vi "Rotation_GetSin.vi"(11 "in ROTATION":T1={"VALUE"=0.0, "COS"=1.0, "SIN"=0.0}) -> (3 "SINE":dbl)   [LabVIEW 2019, in "Trajectory_Library.lvlib"]
doc: "Returns the sine of the rotation.\n\nParameters:\n - in ROTATION - This ROTATION data structure\n\nReturns:\n - Sine of the ROTATAION"
uses:
  Trajectory_Library.lvlib
  ROTATION2D.ctl
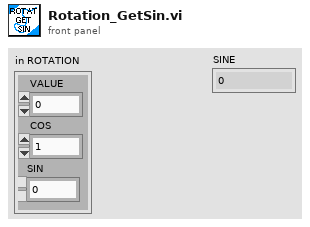
[diagram p1: front panel]
types:
  T1 = typedef "Trajectory_Library.lvlib/ROTATION2D.ctl" = cluster{"VALUE":dbl, "COS":dbl, "SIN":dbl}
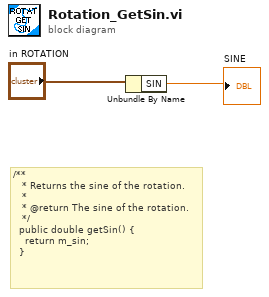
[diagram p0: block diagram]
diagram:
  # "/**\n   * Returns the sine of the rotation.\n   *\n   * @return The sine of the rotation.\n   */\n  public double getSin() {\n    return m_sin;\n  }"
  n1 = Unbundle By Name("in ROTATION") -> ("SIN"=→"SINE":dbl)
